vi "IEEE_754.vi"(11 "input":string) -> (3 "Return":sgl)   [LabVIEW 2015]
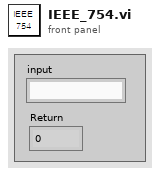
[diagram p1: front panel]
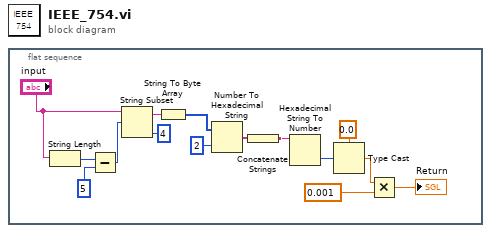
[diagram p0: block diagram]
diagram:
  n1 = flat-sequence {
    frame #0 {
      n2 = String Length(string="input") -> (length=w9:i32)
      n3 = Subtract(x=w9, y=5) -> (x-y=w7:i32)
      n4 = String Subset(string="input", offset (0)=w7, length (rest)=4 ("길이(나머지)")) -> (substring=w4:string)
      n5 = String To Byte Array(string=w4) -> (unsigned byte array=w15:u8[])
      n6 = Number To Hexadecimal String(1:i16 2 ("폭(-)"), 2:w15) -> (0:w12:string[])
      n7 = Concatenate Strings(w12) -> (w11:string)
      n8 = Hexadecimal String To Number(string=w11) -> (number=w13:u32)  [unwired: 2 in, 1 out]
      n9 = Type Cast(type=sgl 0.0, x=w13) -> (*(type *) &x=w2:sgl)
      n10 = Multiply(x=w2, y=0.001) -> (x*y=→"Return":dbl)
    }
  }
